vi "Write Occurrence Ref.vi"(8 "error in (no error)":errorcluster, 10 "Occurrence Ref":refnum<k4>, 11 "Without Data in":refnum<class "Without Data.lvclass">) -> (0 "error out":errorcluster, 3 "Without Data out":refnum<class "Without Data.lvclass">)   [LabVIEW 2020, in "Without Data.lvclass"]
doc: "This VI is used to write the happening of occurrence to the DVR"
uses:
  Classes/Children/Intra-Application/Children/Without data/Without Data.lvclass
  Classes/Children/Intra-Application/Children/Without data/Without Data.lvclass/Without Data.ctl
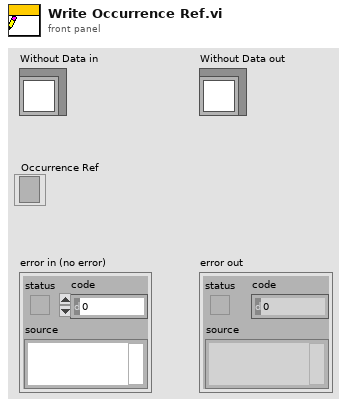
[diagram p1: front panel]
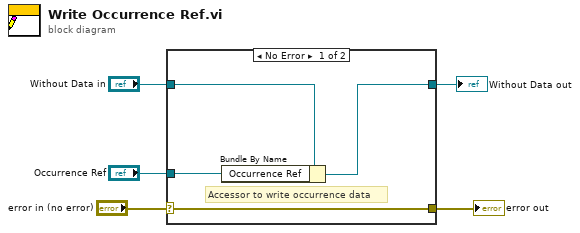
[diagram p0: block diagram]
diagram:
  n1 = case shown="No Error" "error in (no error)" {
    selector: "error in (no error)" -> [w9 w10]
    tunnel: [w9 w10] -> w4
    tunnel: [w7 w11] -> w2
    tunnel: "Without Data in" -> [w8 w11]
    tunnel: "Occurrence Ref" -> [w6 _]
    frame No Error {
      # "Accessor to write occurrence data"
      n2 = Bundle By Name(cluster=w8, "Occurrence Ref"=w6) -> (w7:refnum<class "Without Data.lvclass">)
    }
    frame Error {
    }
  }
  "error out" <- w4
  "Without Data out" <- w2
